vi "Boatx rudder steer.vi"() -> ()   [LabVIEW 2012]
uses:
  <vilib>/Utility/inputDevices.llb/closeKeyboard.vi
  <vilib>/Utility/inputDevices.llb/keyboardAcquire.vi
panel:
  out "IR Volts":dbl
  in  "ESTOP":bool
  in  "Step Size":i32=5
  in  "PC Status":i32=1
  in  "Pan Camera":i32(slide)=1500 scale=500.0..2500.0
  out "Motors Speed":i32(knob) scale=500.0..2500.0
  out "Rudders Direction":i32(knob) scale=500.0..2500.0
  in  "Balance motors":i32(slide) scale=-200.0..200.0
  out "Starboard\nMotor":i32
  out "Port\nMotor":i32
  in  "Balance Rudders":i32(slide) scale=-200.0..200.0
  out "Right\nRubber":i32
  out "Left\nRudder":i32
  out "String Received":string
  out "return count":u32
  out "bytes written":u32
  out "Blinky":bool
  in  "String":string="$CS1500P1500R1500L1500P1500H   1\n"
  in  "stop":bool
  in  "VISA resource name":refnum<visa-resource-name>="COM6"
  # "USE THE ARROW KEYS TO CHANGE THE MOTOR SPEED AND RUDDER POSITION"
  # "DRAG THE SLIDERS TO BALANCE THE MOTOR SPEEDS, BALANCE THE RUDDER ANGLES AND PAN THE CAMERA."
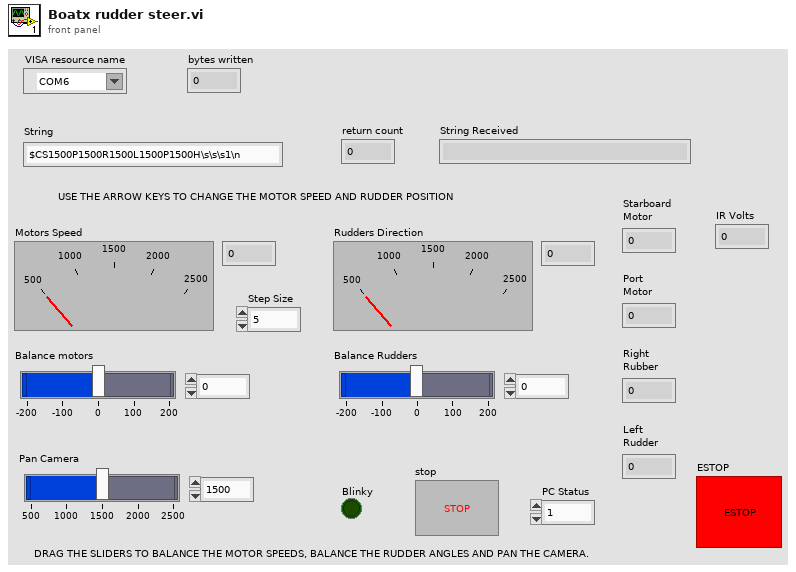
[diagram p1: front panel]
types:
  T1 = enum16{"0", "1", "2", "3", "4", "5", "6", "7", "8", "9", "A", "B", "C", "D", "E", "F", "G", "H", "I", "J", "K", "L", "M", "N", "O", "P", "Q", "R", "S", "T", "U", "V", "W", "X", "Y", "Z", "F1", "F2", "F3", "F4", "F5", "F6", "F7", "F8", "F9", "F10", "F11", "F12", "F13", "F14", "F15", "ADD", "BACK", "BACKSLASH", "CAPITAL", "COMMA", "DECIMAL", "DELETE", "DIVIDE", "DOWN", "END", "EQUALS", "ESCAPE", "GRAVE (`)", "HOME", "INSERT", "LBRACKET", "LCONTROL", "LEFT", "L ALT", "LSHIFT", "LWIN", "MINUS", "MULTIPLY", "NEXT", "NUMLOCK", "NUMPAD_0", "NUMPAD_1", "NUMPAD_2", "NUMPAD_3", "NUMPAD_4", "NUMPAD_5", "NUMPAD_6", "NUMPAD_7", "NUMPAD_8", "NUMPAD_9", "PAUSE", "PERIOD", "PRIOR (PG UP)", "RBRACKET", "RCONTROL", "RETURN", "RIGHT", "R ALT", "RSHIFT", "RWIN", "SCROLL", "SEMICOLON", "SLASH", "SPACE", "SUBTRACT", "TAB", "UP", "ENTER (num pad)", "' (quote)"}[]
  T2 = enum16{"0", "1", "2", "3", "4", "5", "6", "7", "8", "9", "A", "B", "C", "D", "E", "F", "G", "H", "I", "J", "K", "L", "M", "N", "O", "P", "Q", "R", "S", "T", "U", "V", "W", "X", "Y", "Z", "F1", "F2", "F3", "F4", "F5", "F6", "F7", "F8", "F9", "F10", "F11", "F12", "F13", "F14", "F15", "ADD", "BACK", "BACKSLASH", "CAPITAL", "COMMA", "DECIMAL", "DELETE", "DIVIDE", "DOWN", "END", "EQUALS", "ESCAPE", "GRAVE (`)", "HOME", "INSERT", "LBRACKET", "LCONTROL", "LEFT", "L ALT", "LSHIFT", "LWIN", "MINUS", "MULTIPLY", "NEXT", "NUMLOCK", "NUMPAD_0", "NUMPAD_1", "NUMPAD_2", "NUMPAD_3", "NUMPAD_4", "NUMPAD_5", "NUMPAD_6", "NUMPAD_7", "NUMPAD_8", "NUMPAD_9", "PAUSE", "PERIOD", "PRIOR (PG UP)", "RBRACKET", "RCONTROL", "RETURN", "RIGHT", "R ALT", "RSHIFT", "RWIN", "SCROLL", "SEMICOLON", "SLASH", "SPACE", "SUBTRACT", "TAB", "UP", "ENTER (num pad)", "' (quote)"}
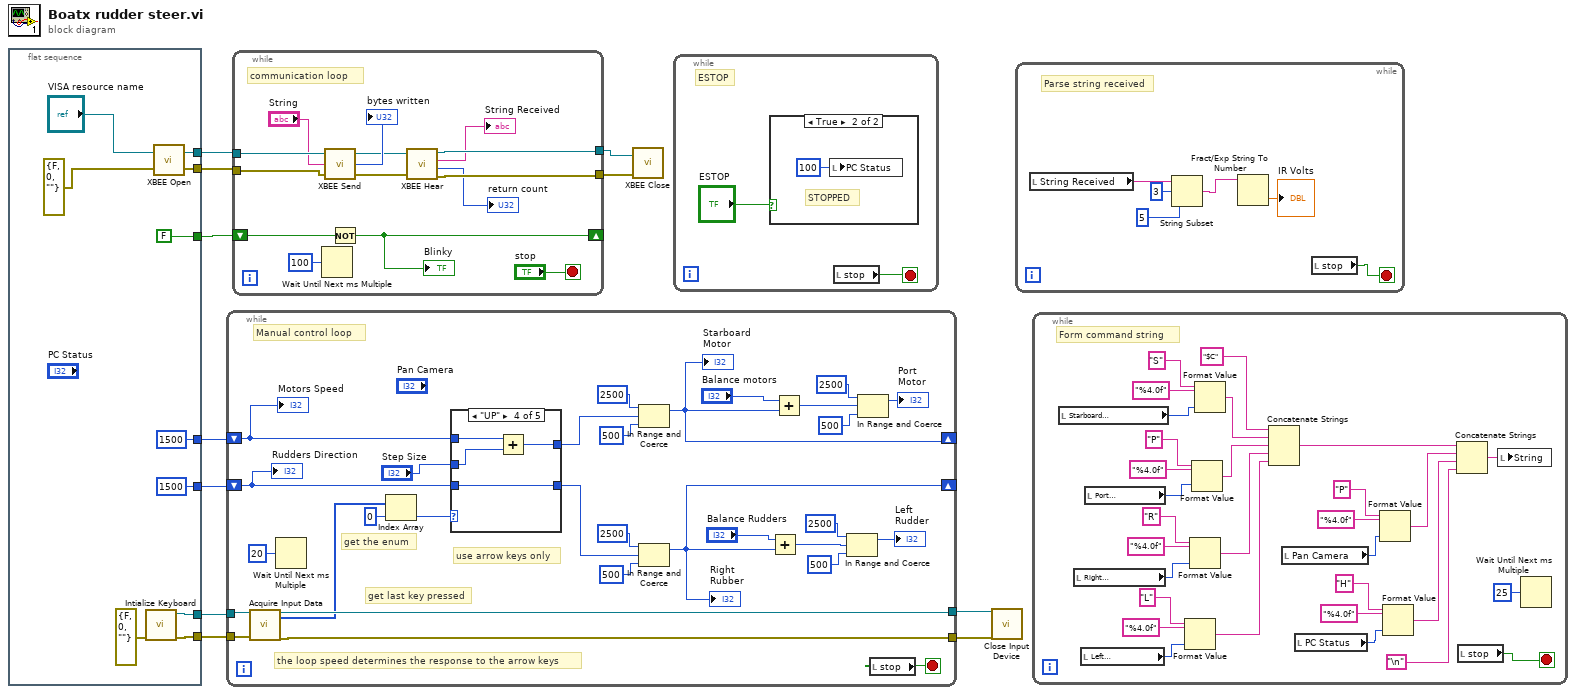
[diagram p0: block diagram]
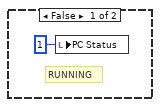
[diagram p2: hidden frame]
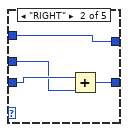
[diagram p4: hidden frame]
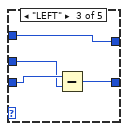
[diagram p5: hidden frame]
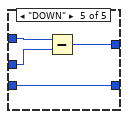
[diagram p6: hidden frame]
diagram:
  n1 = flat-sequence {
    tunnel: [w21] -> w11
    tunnel: [w20] -> w10
    tunnel: [FALSE] -> w7
    tunnel: [w18] -> w6
    tunnel: [w16] -> w5
    tunnel: [1500] -> w2
    tunnel: [1500] -> w1
    frame #0 {
      n2 = call <vilib>:"Intialize Keyboard.vi"("error in (no error)"=errorcluster {"status"=FALSE, "code"=0, "source"=""}) -> ("error out"=w18:errorcluster, "device ID"=w16:refnum<k1>)  [unwired: 9 in]
      n3 = call "XBEE Open.vi"("error in"=errorcluster {"status"=FALSE, "code"=0, "source"=""}, "VISA resource name"="VISA resource name") -> ("error out"=w20:errorcluster, "VISA resource name out"=w21:refnum<visa-resource-name>)
    }
  }
  n4 = while {
    tunnel: w6 -> [w51]
    tunnel: w5 -> [w50]
    tunnel: [w49] -> w4
    tunnel: [w48] -> w3
    shift-right: [w34] -> _
    shift-left: w1 -> [w43]
    shift-right: [w32] -> _
    shift-left: w2 -> [w42]
    stop <- w23 stop-if-true
    # "use arrow keys only"
    # "Manual control loop"
    # "get the enum"
    # "the loop speed determines the response to the arrow keys"
    # "get last key pressed"
    n5 = call-poly <vilib>:"Acquire Input Data.vi"("device ID"=w50, "error in (no error)"=w51) -> ("device ID"=w48:refnum<k1>, "keys pressed"=w47:T1, "error out"=w49:errorcluster)  [unwired: 15 in]
    n6 = Wait Until Next ms Multiple(millisecond multiple=u32 20) -> ()  [unwired: 1 out]
    n7 = Index Array(array=w47, index=0) -> (element=w45:T2)
    n8 = case shown="\"UP\"" w45 {
      tunnel: w43 -> [w53 w57 w61 w63 w67]
      tunnel: [w53 w57 w61 w64 w68] -> w41
      tunnel: w42 -> [w52 w56 w59 w65 w69]
      tunnel: [w52 w55 w60 w65 w69] -> w36
      tunnel: "Step Size" -> [_ w54 w58 w62 w66]
      frame "0", Default {
      }
      frame "RIGHT" {
        n9 = Add(x=w56, y=w54) -> (x+y=w55:i32)
      }
      frame "LEFT" {
        n10 = Subtract(x=w59, y=w58) -> (x-y=w60:i32)
      }
      frame "UP" {
        n11 = Add(x=w63, y=w62) -> (x+y=w64:i32)
      }
      frame "DOWN" {
        n12 = Subtract(x=w67, y=w66) -> (x-y=w68:i32)
      }
    }
    n13 = In Range and Coerce(upper limit=2500, x=w41, lower limit=500) -> (coerced(x)=w34:i32)  [unwired: 1 out]
    "Starboard\nMotor" <- w34
    n14 = In Range and Coerce(upper limit=2500, x=w36, lower limit=500) -> (coerced(x)=w32:i32)  [unwired: 1 out]
    "Right\nRubber" <- w32
    n15 = Add(x="Balance Rudders", y=w32) -> (x+y=w25:i32)
    n16 = Add(x="Balance motors", y=w34) -> (x+y=w29:i32)
    n17 = In Range and Coerce(upper limit=2500, x=w25, lower limit=500) -> (coerced(x)=→"Left\nRudder":i32)  [unwired: 1 out]
    n18 = In Range and Coerce(upper limit=2500, x=w29, lower limit=500) -> (coerced(x)=→"Port\nMotor":i32)  [unwired: 1 out]
    n19 = local read "stop"() -> (w23:bool)
    "Motors Speed" <- w43
    "Rudders Direction" <- w42
  }
  n20 = while {
    tunnel: w11 -> [w82]
    tunnel: w10 -> [w81]
    tunnel: [w76] -> w9
    tunnel: [w75] -> w8
    shift-right: [w79] -> _
    shift-left: w7 -> [w80]
    stop <- "stop" stop-if-true
    # "communication loop"
    n21 = Wait Until Next ms Multiple(millisecond multiple=u32 100) -> ()  [unwired: 1 out]
    n22 = call "XBEE Send.vi"("error in (no error)"=w81, "String"="String", "VISA resource name"=w82) -> ("error out"=w71:errorcluster, "return count"=→"bytes written":u32, "VISA resource name out"=w72:refnum<visa-resource-name>)
    n23 = Not(x=w80) -> (.not. x?=w79:bool)
    "Blinky" <- w79
    n24 = call "XBEE Hear.vi"("VISA resource name"=w72, "error in (no error)"=w71) -> ("VISA resource name out"=w76:refnum<visa-resource-name>, "String Received"=→"String Received":string, "return count"=→"return count":u32, "error out"=w75:errorcluster)
  }
  n25 = call "XBEE Close.vi"("error in (no error)"=w8, "VISA resource name"=w9) -> ()
  n26 = while {
    stop <- w85 stop-if-true
    # "ESTOP"
    n27 = case shown="True" "ESTOP" {
      frame False {
        # "RUNNING"
        n28 = local write "PC Status"(1 ("PC Status")) -> ()
      }
      frame True {
        # "STOPPED"
        n29 = local write "PC Status"(100) -> ()
      }
    }
    n30 = local read "stop"() -> (w85:bool)
  }
  n31 = call-poly <vilib>:"Close Input Device.vi"("error in (no error)"=w4, "device ID"=w3) -> ()  [unwired: 8 in, 1 out]
  n32 = while {
    stop <- w90 stop-if-true
    # "Parse string received"
    n33 = local read "String Received"() -> (w93:string)
    n34 = String Subset(string=w93, offset (0)=3, length (rest)=5 ("length (rest)")) -> (substring=w88:string)
    n35 = Fract/Exp String To Number(string=w88) -> (number=→"IR Volts":dbl)  [unwired: 3 in, 1 out]
    n36 = local read "stop"() -> (w90:bool)
  }
  n37 = while {
    stop <- w123 stop-if-true
    # "Form command string"
    n38 = local read "Starboard\nMotor"() -> (w120:i32)
    n39 = local read "Right\nRubber"() -> (w111:i32)
    n40 = local read "Left\nRudder"() -> (w108:i32)
    n41 = local read "Port\nMotor"() -> (w117:i32)
    n42 = Format Value(string ("")="L", format string="%4.0f", value (0)=w108) -> (output string=w106:string)
    n43 = Format Value(string ("")="R", format string="%4.0f", value (0)=w111) -> (output string=w107:string)
    n44 = Format Value(string ("")="P", format string="%4.0f", value (0)=w117) -> (output string=w114:string)
    n45 = Format Value(string ("")="S", format string="%4.0f", value (0)=w120) -> (output string=w115:string)
    n46 = Concatenate Strings("$C", w115, w114, w107, w106) -> (w98:string)
    n47 = local read "Pan Camera"() -> (w102:i32)
    n48 = local read "PC Status"() -> (w99:i32)
    n49 = Format Value(string ("")="P", format string="%4.0f", value (0)=w102) -> (output string=w97:string)
    n50 = Format Value(string ("")="H", format string="%4.0f", value (0)=w99) -> (output string=w96:string)
    n51 = Concatenate Strings(w98, w97, w96, "\n") -> (w103:string)
    n52 = local read "stop"() -> (w123:bool)
    n53 = local write "String"(w103) -> ()
    n54 = Wait Until Next ms Multiple(millisecond multiple=u32 25) -> ()  [unwired: 1 out]
  }
